vi "Get Values.vi"(1 "Termination Criteria in":refnum<class "Termination Criteria.lvclass">) -> (0 "Term Criteria":T1)   [LabVIEW 2020, in "g_ar_toolkit.common.lvlib" / "Termination Criteria.lvclass"]
uses:
  Termination Criteria.lvclass
  Termination Criteria Values.ctl
  Termination Criteria.lvclass/Termination Criteria.ctl
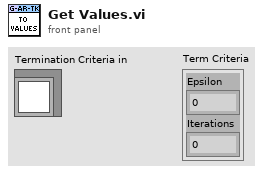
[diagram p1: front panel]
types:
  T1 = typedef "g_ar_toolkit.common.lvlib/Termination Criteria.lvclass/Termination Criteria Values.ctl" = cluster{"Epsilon":dbl, "Iterations":i32}
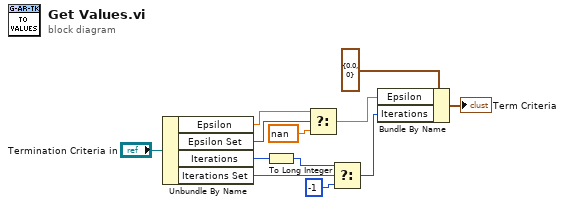
[diagram p0: block diagram]
diagram:
  n1 = Unbundle By Name("Termination Criteria in") -> ("Epsilon"=w6:dbl, "Epsilon Set"=w7:bool, "Iterations"=w10:u16, "Iterations Set"=w11:bool)
  n2 = To Long Integer(number=w10) -> (32bit integer=w9:i32)
  n3 = Select(t=w6, s=w7, f=nan) -> (s? t:f=w2:dbl)
  n4 = Select(t=w9, s=w11, f=-1) -> (s? t:f=w1:i32)
  n5 = Bundle By Name(cluster=T1 {"Epsilon"=0.0, "Iterations"=0} ("Term Criteria"), "Epsilon"=w2, "Iterations"=w1) -> (→"Term Criteria":T1)
